vi "sub_wf_inverse.vi"(11 "Trigger graph":waveform(dbl)(graph)) -> (3 "inverse graph":waveform(dbl)(graph))   [LabVIEW 2016]
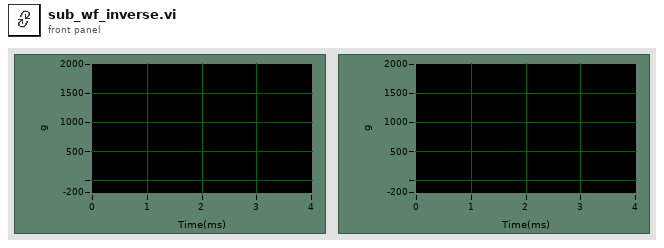
[diagram p1: front panel]
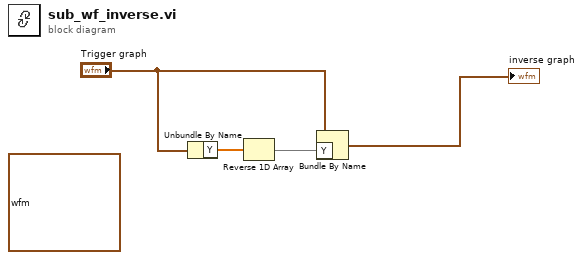
[diagram p0: block diagram]
diagram:
  (unwired) waveform(dbl) {"t0"=timestamp(0 s since 1904-01-01), "dt"=0.00062, "Y"=array[5600 elements]} ("Trigger graph 2")
  n1 = Unbundle By Name("Trigger graph") -> ("Y"=w4:dbl[])
  n2 = Reverse 1D Array(array=w4) -> (reversed array=w3:dbl[])
  n3 = Bundle By Name(cluster="Trigger graph", "Y"=w3) -> (→"inverse graph":waveform(dbl))
